vi "_PC_MS_SubVI setWfmGraphAttr.vi"(8 "error in (no error)":errorcluster, 10 "plotValue":waveform(sgl)[](array[waveform]), 11 "graph in":refnum<vi>) -> (0 "error out":errorcluster, 3 "graph out":refnum<vi>)   [LabVIEW 2018]
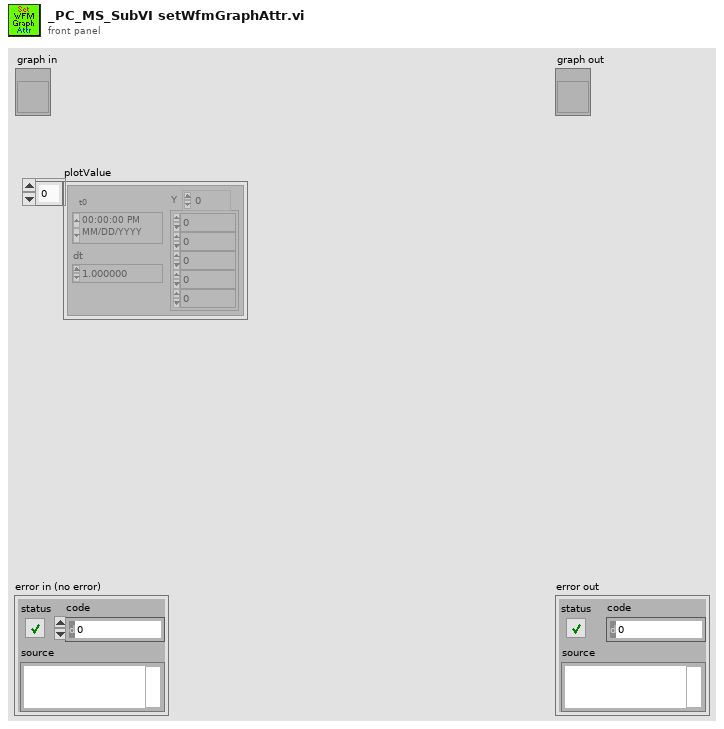
[diagram p1: front panel]
types:
  T1 = cluster{"BGColor":u32, "GridX":bool, "GridY":bool, "LineColorArray":u32[], "LineWidthArray":u8[]}
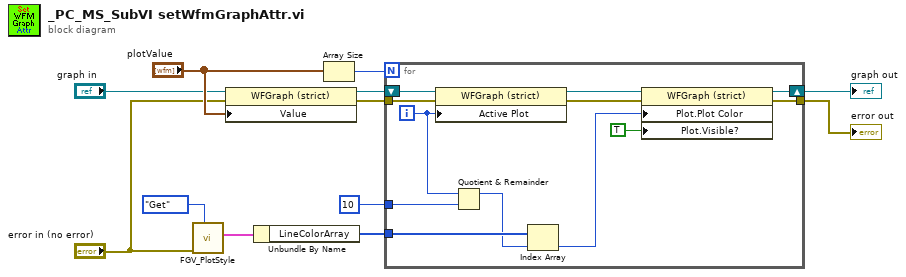
[diagram p0: block diagram]
diagram:
  n1 = call "FGV_PlotStyle.vi"("Function"=enum16{"Set", "Get"}."Get", "error in (no error)"="error in (no error)") -> ("Output Cluster"=w11:T1)  [unwired: 8 in, 1 out]
  n2 = property class="WFGraph (strict)"(reference="graph in", error in="error in (no error)", "Value"="plotValue") -> (reference out=w1:refnum<vi>, error out=w2:errorcluster)
  n3 = Unbundle By Name(w11) -> ("LineColorArray"=w10:u32[])
  n4 = Array Size(array="plotValue") -> (size(s)=w3:i32)
  n5 = for {
    N: w3 -> [_]
    tunnel: [w22] -> w8
    tunnel: w10 -> [w18]
    tunnel: 10 -> [w19]
    tunnel: w2 -> [w15]
    shift-right: [w13] -> w6
    shift-left: w1 -> [w24]
    i -> [w20]
    n6 = property class="WFGraph (strict)"(reference=w24, error in=w15, "Active Plot"=w20) -> (reference out=w23:refnum<vi>, error out=w21:errorcluster)
    n7 = Quotient & Remainder(x=w20, y=w19) -> (x-y*floor(x/y)=w16:i32)  [unwired: 1 out]
    n8 = Index Array(array=w18, index=w16) -> (element=w17:u32)
    n9 = property class="WFGraph (strict)"(reference=w23, error in=w21, "Plot.Plot Color"=w17, "Plot.Visible?"=TRUE ("Plot.Visible")) -> (reference out=w13:refnum<vi>, error out=w22:errorcluster)
  }
  "error out" <- w8
  "graph out" <- w6
